vi "Dequeue.vi"(8 "error in (no error)":errorcluster, 11 "Queue in":refnum<queue>) -> (0 "error out":errorcluster, 1 "Dato":variant, 3 "Mensaje":string)   [LabVIEW 2018, in "Mensajes.lvlib"]
uses:
  Controles/Mensaje Data.ctl
  Mensajes.lvlib
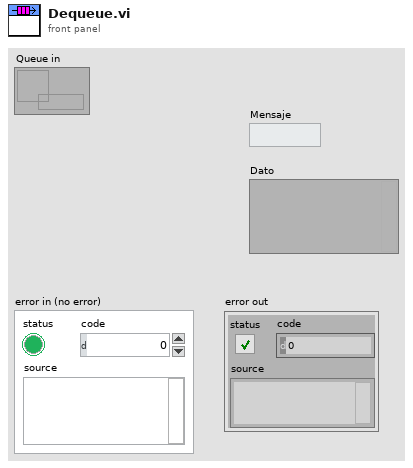
[diagram p1: front panel]
types:
  T1 = typedef "Mensaje Data.ctl" = cluster{"Mensaje":string, "Dato":variant}
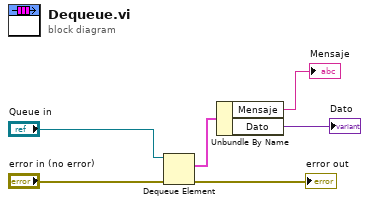
[diagram p0: block diagram]
diagram:
  n1 = Dequeue Element(queue="Queue in", error in (no error)="error in (no error)") -> (element=w3:T1, error out=→"error out":errorcluster)  [unwired: 1 in, 2 out]
  n2 = Unbundle By Name(w3) -> ("Mensaje"=→"Mensaje":string, "Dato"=→"Dato":variant)
